vi "Reserve Aquirer.vi"(8 "error in (no error)":errorcluster, 11 "Instrument Handler in":refnum<class "Instrument Handler.lvclass">) -> (0 "error out":errorcluster, 1 "Aquirer Index":i32, 2 "Aquirer":T1, 3 "Instrument Handler out":refnum<class "Instrument Handler.lvclass">)   [LabVIEW 2020, in "Instrument Handler.lvlib" / "Instrument Handler.lvclass"]
doc: "Reserve an Aquirer from the Instrument Handler. Create new Aquirer if no Aquirers are available."
uses:
  Instrument Handler.lvclass
  Controls/Ctl_AquirerRefnum.ctl
  Instrument Handler.lvclass/Instrument Handler.ctl
  Controls/Ctl_AquirerAvailabilityStatus.ctl
  Instrument Handler.lvlib
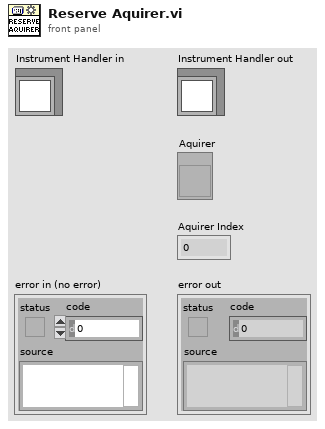
[diagram p1: front panel]
types:
  T1 = typedef "Instrument Handler.lvlib/Ctl_AquirerRefnum.ctl" = refnum<vi>
  T2 = typedef "Instrument Handler.lvlib/Ctl_AquirerAvailabilityStatus.ctl" = cluster{"Available?":bool, "Aquirer":T1}
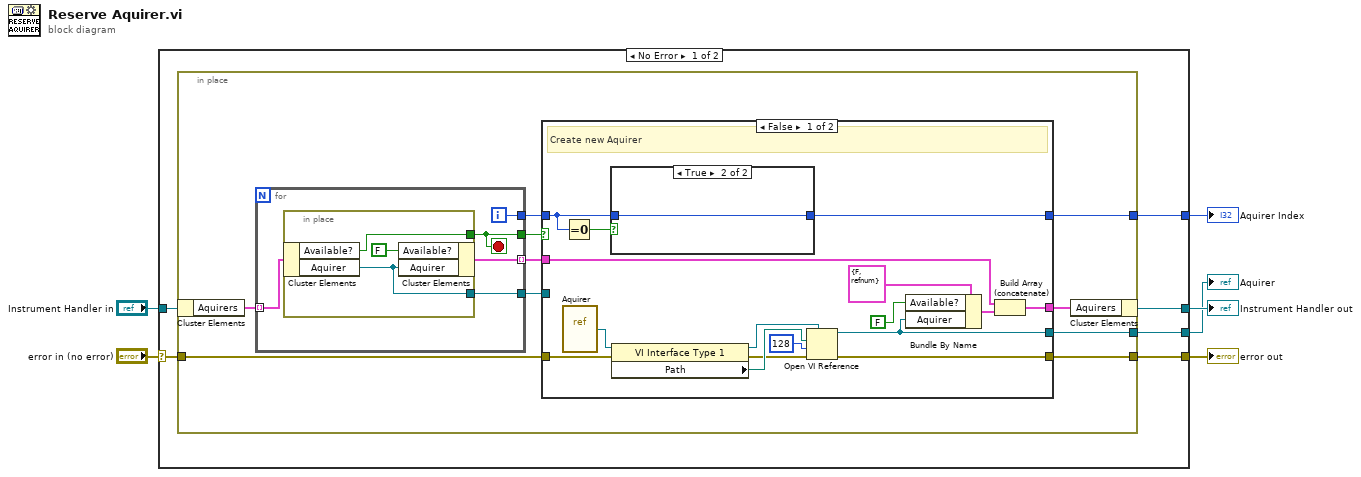
[diagram p0: block diagram]
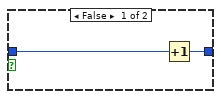
[diagram p2: hidden frame]
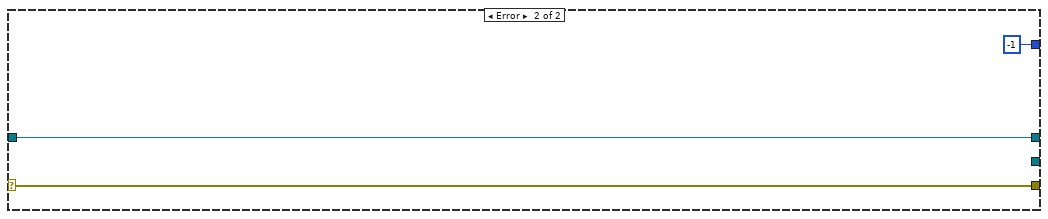
[diagram p4: hidden frame]
diagram:
  n1 = case shown="No Error" "error in (no error)" {
    selector: "error in (no error)" -> [w8 w56]
    tunnel: [w7 w56] -> w5
    tunnel: [w9 w55] -> w3
    tunnel: "Instrument Handler in" -> [w12 w55]
    tunnel: [w11 _] -> w2
    tunnel: [w10 -1] -> w1
    frame No Error {
      n2 = in-place {
        in-place-border: [w15] -> w11
        in-place-border: [w17] -> w10
        in-place-border: w8 -> [w18]
        in-place-border: [w13] -> w7
        n3 = in-place-cluster #1(w12) -> ("Aquirers"=w22:T2[])
        n4 = for {
          tunnel: w22 -> [w50] mode=indexing
          tunnel: [w49] -> w19 mode=indexing
          tunnel: [w48] -> w21
          tunnel: [w47] -> w14
          tunnel: [w46] -> w16
          i -> [w46]
          stop <- w48 stop-if-true
          n5 = in-place {
            in-place-border: [w52] -> w48
            in-place-border: [w51] -> w47
            n6 = in-place-cluster #2(w50) -> ("Available?"=w52:bool, "Aquirer"=w51:T1)
            n7 = in-place-cluster #2("Available?"=FALSE, "Aquirer"=w51) -> (w49:T2)
          }
        }
        n8 = case shown="False" w21 {
          tunnel: [w25 w45] -> w20
          tunnel: w19 -> [w27 w45]
          tunnel: w18 -> [w36 w42]
          tunnel: [w29 w44] -> w17
          tunnel: w16 -> [w24 w44]
          tunnel: [w28 w43] -> w15
          tunnel: w14 -> [_ w43]
          tunnel: [w30 w42] -> w13
          frame False {
            # "Create new Aquirer"
            n9 = vi-ref "Aquirer.vi"() -> (w38:refnum<vi>)
            n10 = Equal To 0?(x=w24) -> (x = 0?=w23:bool)
            n11 = case shown="True" w23 {
              tunnel: [w40 w41] -> w29
              tunnel: w24 -> [w39 w41]
              frame False {
                n12 = Increment(x=w39) -> (x+1=w40:i32)
              }
              frame True {
              }
            }
            n13 = property class="VI Interface Type 1"(reference=w38, error in=w36) -> (reference out=w33:refnum<vi>, error out=w35:errorcluster, "Path"=w37:path)
            n14 = Open VI Reference(type specifier VI Refnum (for type only)=w33, vi path=w37, options=128, error in (no error)=w35) -> (vi reference=w28:refnum<vi>, error out=w30:errorcluster)  [unwired: 2 in]
            n15 = Bundle By Name(cluster=T2 {"Available?"=FALSE, "Aquirer"=refnum} ("Instrument cluster"), "Available?"=FALSE, "Aquirer"=w28) -> (w26:T2)
            n16 = Build Array (concatenate)(w27, w26) -> (w25:T2[])
          }
          frame True {
            # "Aquirer reserved"
          }
        }
        n17 = in-place-cluster #1("Aquirers"=w20) -> (w9:refnum<class "Instrument Handler.lvclass">)
      }
    }
    frame Error {
    }
  }
  "error out" <- w5
  "Instrument Handler out" <- w3
  "Aquirer Index" <- w1
  "Aquirer" <- w2
